vi "Pivot Module.vi"(0 "Rotational Motor Refnum":string="My Motor RefNum", 1 "Encoder Refnum":string="My AnalogChannel RefNum", 2 "Top Voltage":dbl, 5 "Drive Motor Refnum":string="My Motor RefNum", 9 "Motor Angle":dbl, 11 "Motor Speed":dbl, 12 "Calibration Angle":dbl, 13 "Bottom Voltage":dbl) -> ()   [LabVIEW 2014]
uses:
  <vilib>/Rock Robotics/WPI/SafetyOutput/WPI_SafetyOutputConfigMenu.ctl
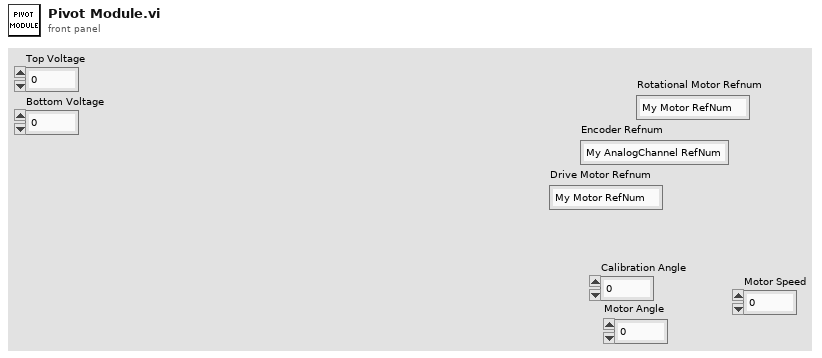
[diagram p1: front panel]
types:
  T1 = typedef "WPI_SafetyOutputConfigMenu.ctl" = enum16{"Enable", "Disable"}
  T2 = typedef "WPI_AnalogChannelDevRef.ctl" = cluster{"DevStatus":errorcluster, "Controller":T3, "Analog Channel":T4}
  T3 = typedef "FPGA_TypedefAnalogModule.ctl" = enum16{"Controller 1"}
  T4 = typedef "FPGA_AIChannel.ctl" = enum8{"AI 0", "AI 1", "AI 2", "AI 3", "AI MXP 0", "AI MXP 1", "AI MXP 2", "AI MXP 3", "Invalid"}
  T5 = typedef "WPI_MotorControlDeviceRef.ctl" = cluster{"DeviceStatus":errorcluster, "Type":T6, "PWM":cluster{"Controller":T7, "PWM Channel":T8, "DeadBand":T9}, "CAN":cluster{"Device Number":u8, "Control Mode":T10, "Semaphore":T11, "Max Vout":dbl, "TalonSRX Control Mode":T12}, "Invert":bool, "TransformRef":T13, "InvTransformRef":T13}
  T6 = typedef "WPI_MotorControlType.ctl" = enum16{"PWM", "CAN", "CANTalonSRX"}
  T7 = typedef "FPGA_TypedefDigitalModule.ctl" = enum16{"Controller 1"}
  T8 = typedef "FPGA_DIOPWMChannel.ctl" = enum8{"PWM 0", "PWM 1", "PWM 2", "PWM 3", "PWM 4", "PWM 5", "PWM 6", "PWM 7", "PWM 8", "PWM 9", "PWM MXP 0", "PWM MXP 1", "PWM MXP 2", "PWM MXP 3", "PWM MXP 4", "PWM MXP 5", "PWM MXP 6", "PWM MXP 7", "PWM MXP 8", "PWM MXP 9", "Invalid"}
  T9 = typedef "WPI_PWMDeadband.ctl" = cluster{"Name":string, "maxPositivePwm":i32, "minPositivePwm":i32, "centerPwm":i32, "maxNegativePwm":i32, "minNegativePwm":i32, "angularRange":u16}
  T10 = typedef "WPI_CANJaguar_ControlMode.ctl" = enum8{"Percent VBus", "Current", "Speed", "Position", "Voltage"}
  T11 = typedef "Semaphore RefNum" = refnum<k1>
  T12 = typedef "WPI_CANTalonSRX_APIControlMode.ctl" = enum8{"Percent VBus", "Speed", "Position", "Slave", "Unchanged / Invalid"}
  T13 = typedef "WPI_PWMTransform_ConPane.ctl" = refnum<vi>
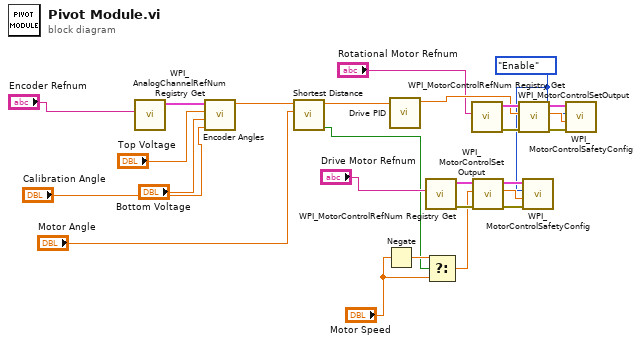
[diagram p0: block diagram]
diagram:
  w8 = WPI_SafetyOutputConfigMenu."Enable" ("mode")
  n1 = call <vilib>:"WPI_AnalogChannelRefNum Registry Get.vi"("refnum name"="Encoder Refnum") -> ("AIDeviceRef"=w25:T2)  [unwired: 9 in, 1 out]
  n2 = call "Encoder Angles.vi"("Calibration Angle"="Calibration Angle", "Bottom Voltage"="Bottom Voltage", "Top Voltage"="Top Voltage", "AIDeviceRef Encoder"=w25) -> ("Encoder Angle"=w23:dbl)  [unwired: 7 in]
  n3 = call "Shortest Distance.vi"("Target"="Motor Angle", "Current"=w23) -> ("Flipping?"=w3:bool, "Angle to Rotate"=w21:dbl)  [unwired: 8 in]
  n4 = Negate(x="Motor Speed") -> (-x=w5:dbl)
  n5 = call "Drive PID.vi"("Process Variable"=w21) -> ("Output"=w10:dbl)  [unwired: 10 in]
  n6 = call <vilib>:"WPI_MotorControlRefNum Registry Get.vi"("refnum name"="Drive Motor Refnum") -> ("error out"=w15:errorcluster, "MotorControlDevRef"=w14:T5)  [unwired: 9 in]
  n7 = Select(t=w5, s=w3, f="Motor Speed") -> (s? t:f=w6:dbl)
  n8 = call <vilib>:"WPI_MotorControlRefNum Registry Get.vi"("refnum name"="Rotational Motor Refnum") -> ("error out"=w20:errorcluster, "MotorControlDevRef"=w19:T5)  [unwired: 9 in]
  n9 = call <vilib>:"WPI_MotorControlSetOutput.vi"("error in (no error)"=w15, "Output"=w6, "MotorControlDevRef"=w14) -> ("error out"=w13:errorcluster, "Motor Output"=w12:dbl, "MotorControlDevRef"=w11:T5)  [unwired: 6 in]
  n10 = call <vilib>:"WPI_MotorControlSetOutput.vi"("error in (no error)"=w20, "Output"=w10, "MotorControlDevRef"=w19) -> ("error out"=w18:errorcluster, "Motor Output"=w17:dbl, "MotorControlDevRef"=w16:T5)  [unwired: 6 in]
  n11 = call <vilib>:"WPI_MotorControlSafetyConfig.vi"("error in (no error)"=w13, "timeout (s)"=w12, "mode"=w8, "MotorControlDevRef"=w11) -> ()  [unwired: 6 in, 2 out]
  n12 = call <vilib>:"WPI_MotorControlSafetyConfig.vi"("error in (no error)"=w18, "timeout (s)"=w17, "mode"=w8, "MotorControlDevRef"=w16) -> ()  [unwired: 6 in, 2 out]
